vi "Module Template SM.vi"(8 "error in (no error)":errorcluster, 11 "Module_Refs":T1={"ModuleName"=enum."Controller", "Queue"=refnum, "user event"=refnum, "VI Refnum"=refnum, "ShowFP"=FALSE, "StatesTracking Enabled"=FALSE}) -> (0 "error out":errorcluster)   [LabVIEW 2019, in "Architecture.lvlib" / "Module Template.lvlib"]
doc: "Main Module Template of the architecture. Use this as a template to integrate new independent processes into your application."
uses:
  Modules/Module Template/Module Template.lvlib
  Typedefs/Module References.ctl
  Typedefs/Enum_Module_Name.ctl
  Typedefs/Message.ctl
  Typedefs/State Machine Data.ctl
  Modules/Module Template/Typedefs/Config.ctl
  Typedefs/Application Configuration.ctl
  Modules/Module Template/SubVIs/Module Template Configuraton Extractor API.vi
  Architecture.lvlib
panel:
  in  "Stop App":bool
  out "Message":string
  in  "Stop Module":bool
  # "#Architecture\n\nPlace inside this box all visible data."
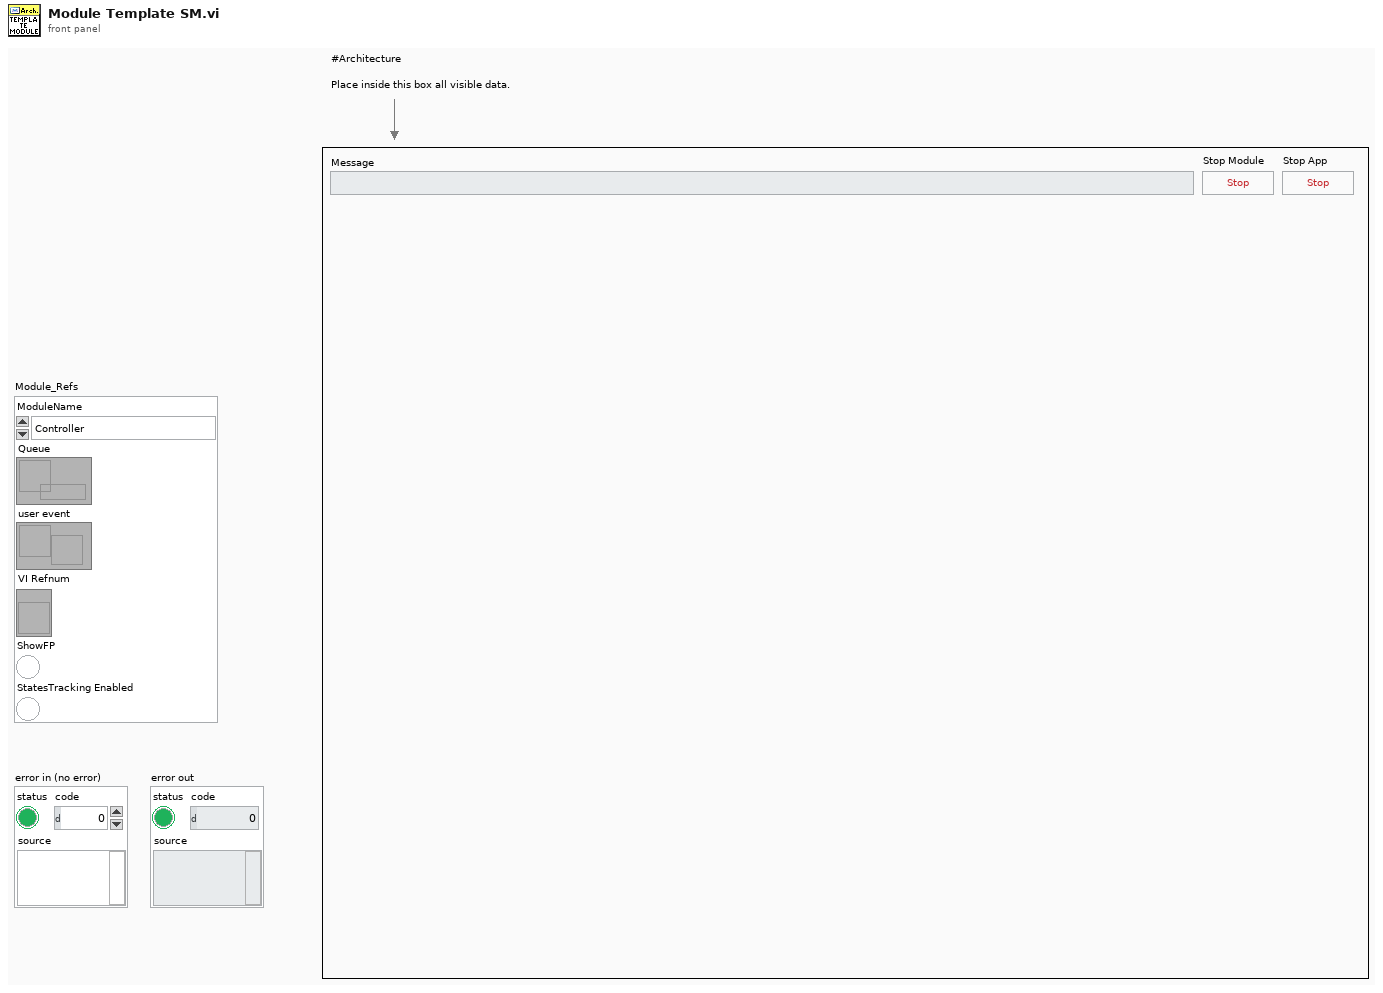
[diagram p1: front panel]
types:
  T1 = typedef "Architecture.lvlib/Module References.ctl" = cluster{"ModuleName":T2, "Queue":refnum<queue>, "user event":refnum<user-event>, "VI Refnum":refnum<vi>, "ShowFP":bool, "StatesTracking Enabled":bool}
  T2 = typedef "Architecture.lvlib/Enum_Module_Name.ctl" = enum16{"Configuration", "Error_Handler", "Log", "Database", "Controller", "User Console", "Display Console", "Sensor Interface"}
  T3 = typedef "Architecture.lvlib/Module Template.lvlib/State Machine Data.ctl" = cluster{"Module_Refs":T1, "Response Data":variant, "Module Template Config":T4}
  T4 = typedef "Architecture.lvlib/Module Template.lvlib/Config.ctl" = cluster{"Module Enabled":bool}
  T5 = enum32{"Invalid", "Standard", "Closed", "Hidden", "Minimized", "Maximized"}
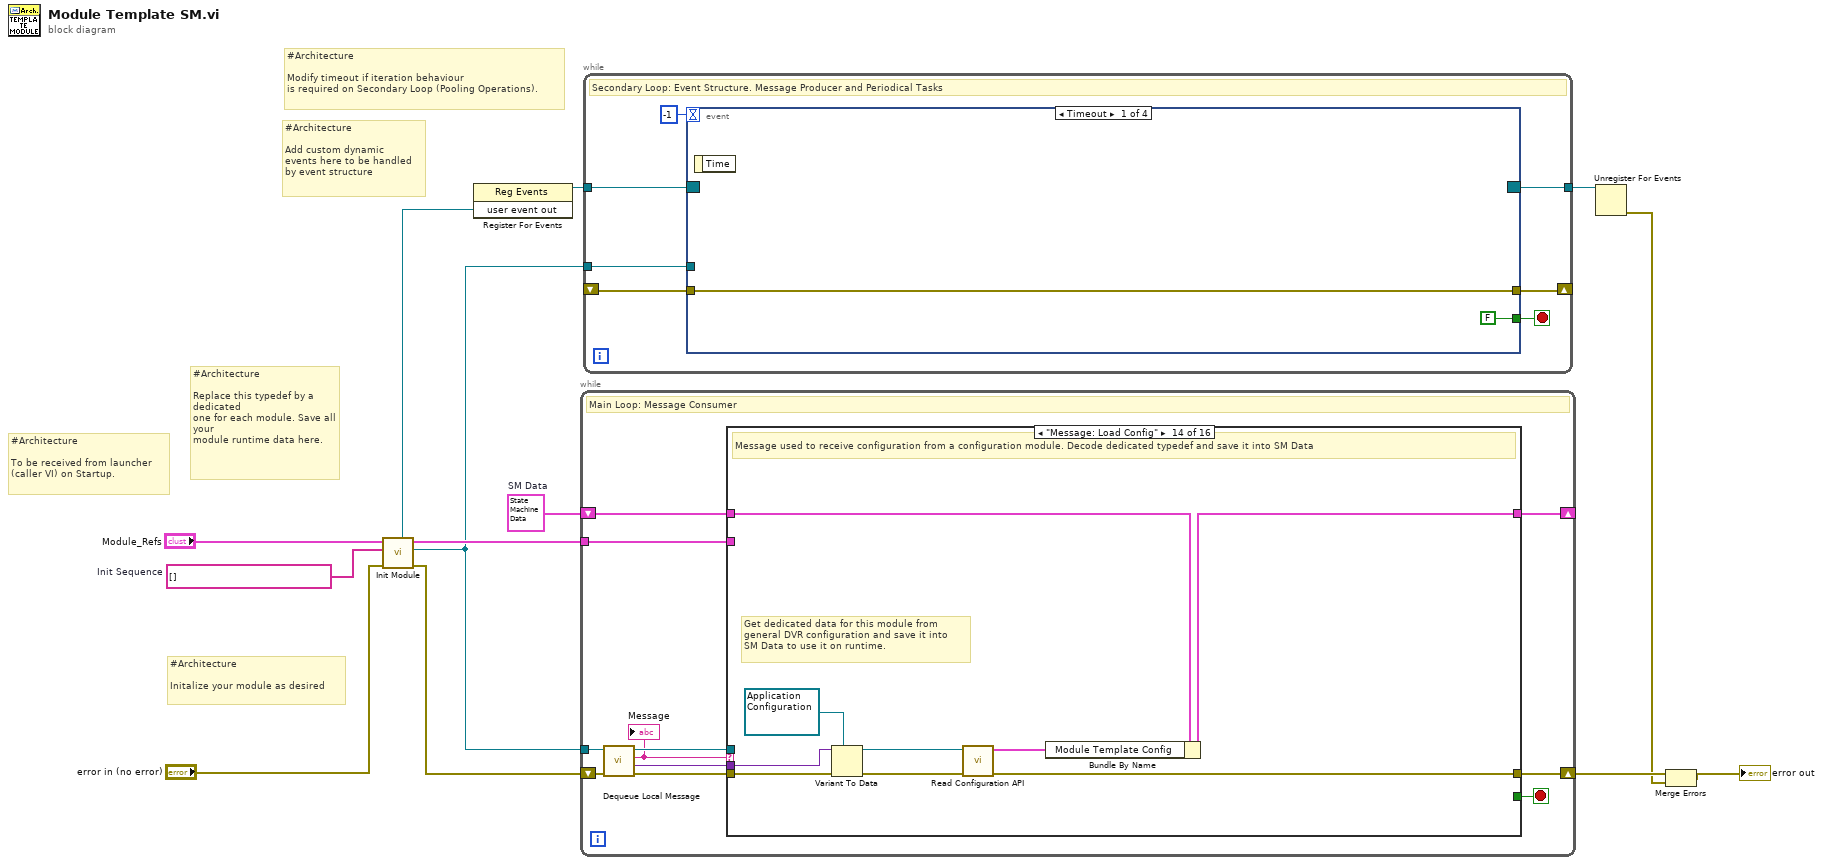
[diagram p0: block diagram]
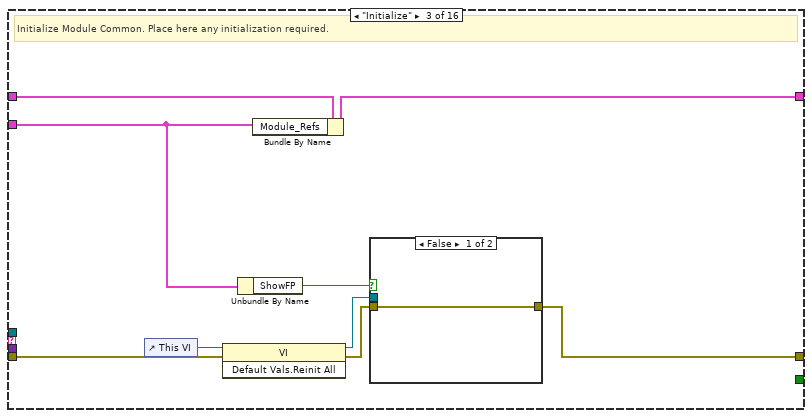
[diagram p4: hidden frame]
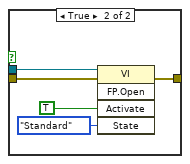
[diagram p5: hidden frame]
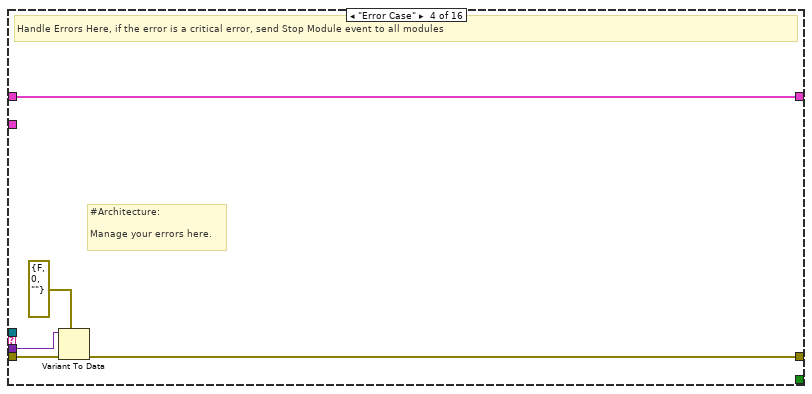
[diagram p6: hidden frame]
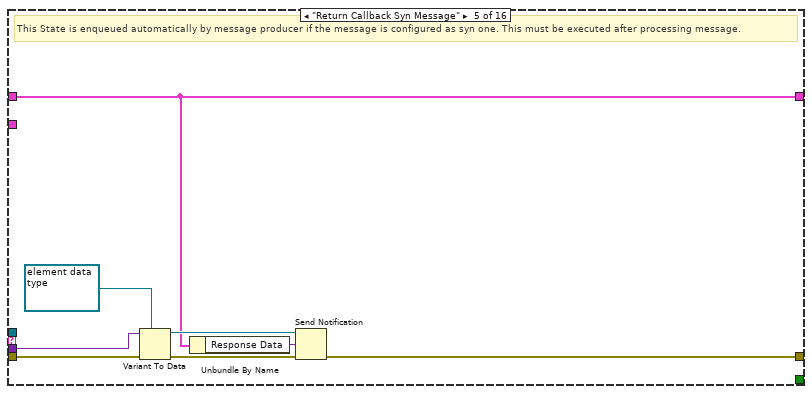
[diagram p7: hidden frame]
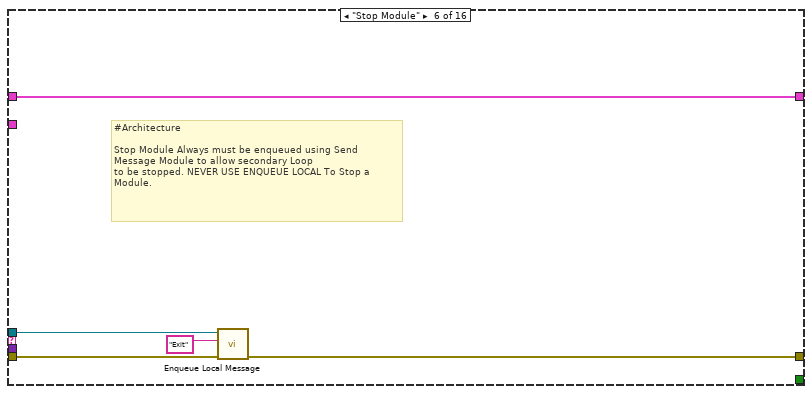
[diagram p8: hidden frame]
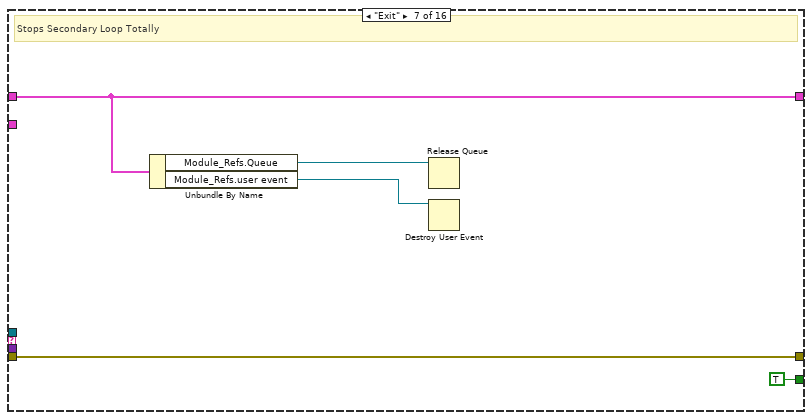
[diagram p9: hidden frame]
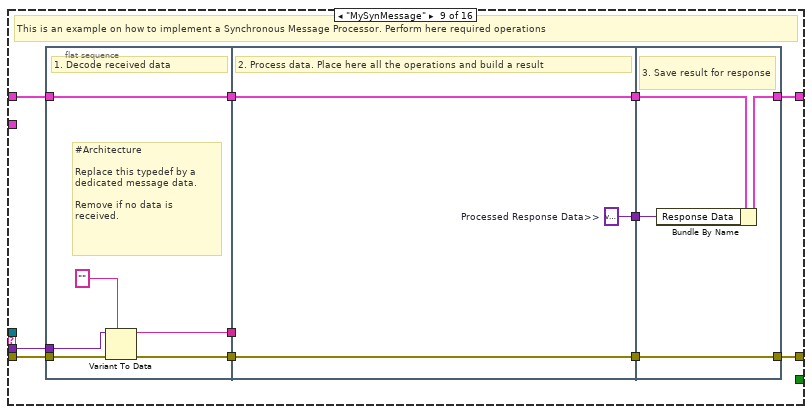
[diagram p11: hidden frame]
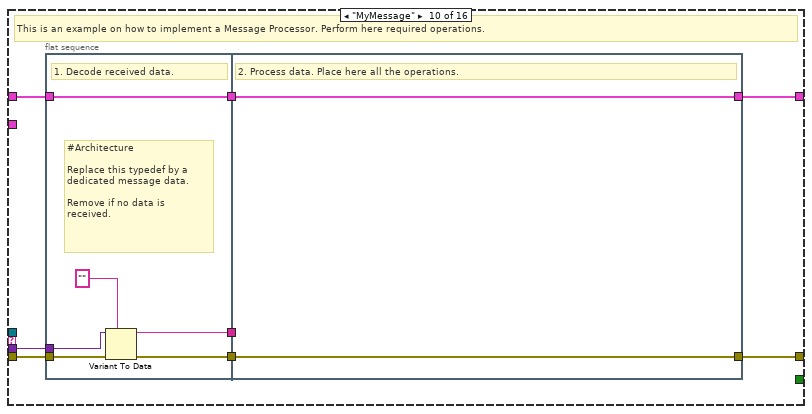
[diagram p12: hidden frame]
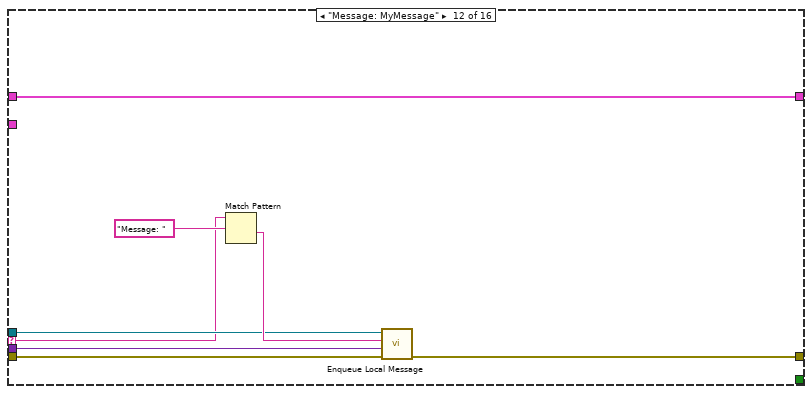
[diagram p14: hidden frame]
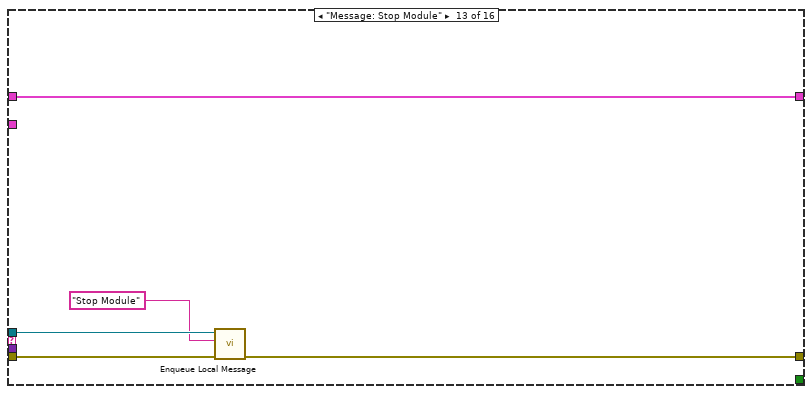
[diagram p15: hidden frame]
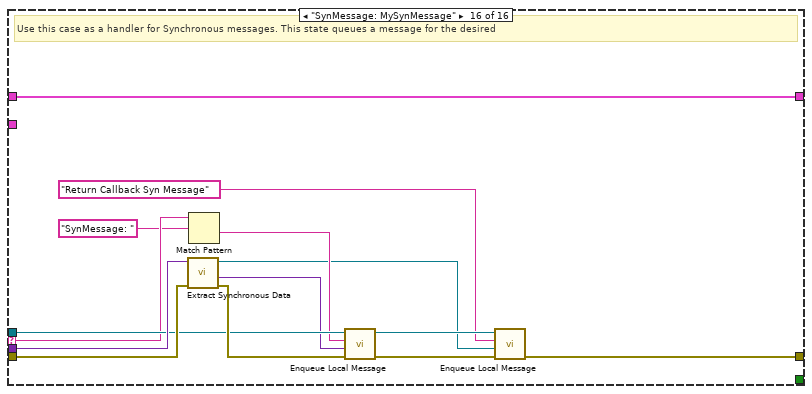
[diagram p17: hidden frame]
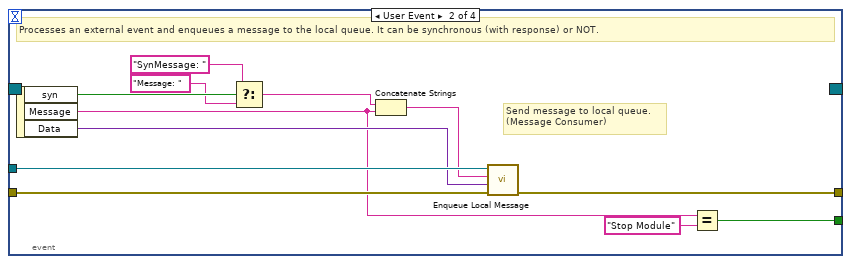
[diagram p18: hidden frame]
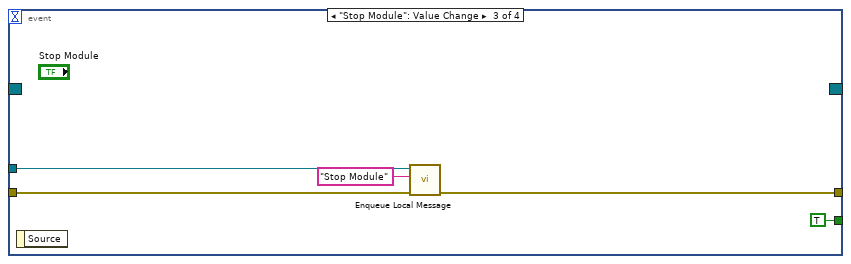
[diagram p19: hidden frame]
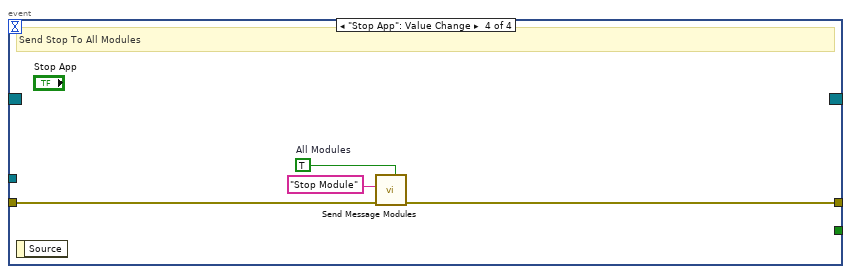
[diagram p20: hidden frame]
diagram:
  w10 = string[] []  # Init Sequence
  w13 = T3 {"Module_Refs"={"ModuleName"=enum."Controller", "Queue"=refnum, "user event"=refnum, "VI Refnum"=refnum, "ShowFP"=FALSE, "StatesTracking Enabled"=FALSE}, "Response Data"=variant, "Module Template Config"={"Module Enabled"=FALSE}}  # SM Data
  # "#Architecture\n\nModify timeout if iteration behaviour \nis required on Secondary Loop (Pooling Operations)."
  # "#Architecture\n\nAdd custom dynamic \nevents here to be handled \nby event structure"
  # "#Architecture\n\nInitalize your module as desired"
  # "#Architecture\n\nTo be received from launcher \n(caller VI) on Startup."
  # "#Architecture\n\nReplace this typedef by a dedicated \none for each module. Save all your \nmodule runtime data here."
  n1 = call "Init Module.vi"("error in (no error)"="error in (no error)", "Init Sequence"=w10, "Module Refs"="Module_Refs") -> ("error out"=w12:errorcluster, "queue out"=w1:refnum<queue>, "Module Refs Out"=w3:T1, "user event out"=w2:refnum<user-event>)  [unwired: 5 in]
  n2 = register-events(w2) -> (reference out=w9:refnum<event-registration>)  [unwired: 2 in, 1 out]
  n3 = while {
    shift-right: [w23] -> _
    shift-left: w13 -> [w24]
    shift-right: [w22] -> w7
    shift-left: w12 -> [w20]
    tunnel: w1 -> [w21]
    tunnel: w3 -> [w14]
    stop <- w15 stop-if-true
    # "Main Loop: Message Consumer"
    n4 = call "Dequeue Local Message.vi"("error in"=w20, "Msg queue in"=w21) -> ("error out"=w19:errorcluster, "Data"=w16:variant, "Message"=w17:string, "queue out"=w18:refnum<queue>)  [unwired: 6 in]
    "Message" <- w17
    n5 = case shown="\"Message: Load Config\"" w17 {
      selector: w17 -> [_ _ _ _ _ _ _ _ _ _ _ w111 _ _ _ w143]
      tunnel: w24 -> [w26 w28 w37 w48 w50 w61 w64 w68 w79 w100 w110 w118 w123 w132 w134 w148]
      tunnel: [w26 w28 w35 w48 w50 w61 w64 w68 w78 w93 w110 w118 w123 w125 w134 w148] -> w23
      tunnel: w19 -> [w25 w27 w36 w47 w56 w60 w66 w67 w72 w96 w109 w115 w122 w131 w133 w147]
      tunnel: [w25 w27 w31 w46 w55 w59 w66 w67 w77 w99 w109 w112 w121 w126 w133 w137] -> w22
      tunnel: w18 -> [_ _ _ _ _ w58 _ _ _ _ _ w113 w120 _ _ w144]
      tunnel: w16 -> [_ _ _ w45 w53 _ _ _ w71 w95 _ w114 _ w130 _ w145]
      tunnel: [_ _ _ _ _ _ TRUE _ _ _ _ _ _ _ _ _] -> w15
      tunnel: w14 -> [_ _ w34 _ _ _ _ _ _ _ _ _ _ _ _ _]
      frame "--------State Machine Arquitechture Operations--------" {
      }
      frame "Idle", Default {
        # "Use this state to make iterations if required."
      }
      frame "Initialize" {
        # "Initialize Module Common. Place here any initialization required."
        n6 = control-ref of="This VI"() -> (w29:refnum<vi>)
        n7 = invoke class="VI" method="Default Vals.Reinit All"(reference=w29, error in=w36) -> (reference out=w32:refnum<vi>, error out=w33:errorcluster)  [unwired: 1 in, 1 out]
        n8 = Unbundle By Name(w34) -> ("ShowFP"=w30:bool)
        n9 = Bundle By Name(cluster=w37, "Module_Refs"=w34) -> (w35:T3)
        n10 = case shown="False" w30 {
          tunnel: w33 -> [w38 w43]
          tunnel: [w38 w42] -> w31
          tunnel: w32 -> [_ w41]
          frame False {
          }
          frame True {
            n11 = invoke class="VI" method="FP.Open"(reference=w41, error in=w43, "Activate"=TRUE ("Activate?"), "State"=T5."Standard") -> (error out=w42:errorcluster)  [unwired: 1 in, 4 out]
          }
        }
      }
      frame "Error Case" {
        # "#Architecture: \n\nManage your errors here."
        # "Handle Errors Here, if the error is a critical error, send Stop Module event to all modules"
        n12 = Variant To Data(error in=w47, type=errorcluster {"status"=FALSE, "code"=0, "source"=""} ("error constant"), Variant=w45) -> (error out=w46:errorcluster)  [unwired: 1 out]
      }
      frame "Return Callback Syn Message" {
        # "This State is enqueued automatically by message producer if the message is configured as syn one. This must be executed after processing message."
        n13 = Variant To Data(error in=w56, type=refnum<notifier> refnum ("notifier out"), Variant=w53) -> (data=w51:refnum<notifier>, error out=w54:errorcluster)
        n14 = Unbundle By Name(w50) -> ("Response Data"=w49:variant)
        n15 = Send Notification(notification=w49, notifier=w51, error in (no error)=w54) -> (error out=w55:errorcluster)  [unwired: 1 out]
      }
      frame "Stop Module" {
        # "#Architecture\n\nStop Module Always must be enqueued using Send Message Module to allow secondary Loop\nto be stopped. NEVER USE ENQUEUE LOCAL To Stop a Module."
        n16 = call "Enqueue Local Message.vi"("error in"=w60, "Message"="Exit", "Msg queue in"=w58) -> ("error out"=w59:errorcluster)  [unwired: 7 in, 1 out]
      }
      frame "Exit" {
        # "Stops Secondary Loop Totally"
        n17 = Unbundle By Name(w64) -> ("Module_Refs.Queue"=w63:refnum<queue>, "Module_Refs.user event"=w62:refnum<user-event>)
        n18 = Release Queue(queue=w63) -> ()  [unwired: 2 in, 3 out]
        n19 = Destroy User Event(user event=w62) -> ()  [unwired: 1 in, 1 out]
      }
      frame "--------------State Machine Custom States-------------" {
      }
      frame "MySynMessage" {
        # "This is an example on how to implement a Synchronous Message Processor. Perform here required operations"
        n20 = flat-sequence {
          tunnel: w72 -> [w83]
          tunnel: w79 -> [w85]
          tunnel: [w85] -> w76
          tunnel: [w81] -> w75
          tunnel: w71 -> [w82]
          tunnel: [w80] -> w70
          tunnel: w76 -> [w88]
          tunnel: w75 -> [w87]
          tunnel: [w88] -> w74
          tunnel: [w87] -> w73
          tunnel: w70 -> [_]
          tunnel: [w86] -> w69
          tunnel: [w91] -> w77
          tunnel: [w90] -> w78
          tunnel: w74 -> [w92]
          tunnel: w73 -> [w91]
          tunnel: w69 -> [w89]
          frame #0 {
            # "#Architecture\n\nReplace this typedef by a dedicated message data.\n\nRemove if no data is received."
            # "1. Decode received data"
            n21 = Variant To Data(error in=w83, type="", Variant=w82) -> (data=w80:string, error out=w81:errorcluster)
          }
          frame #1 {
            w86 = variant  # Processed Response Data>>
            # "2. Process data. Place here all the operations and build a result"
          }
          frame #2 {
            # "3. Save result for response"
            n22 = Bundle By Name(cluster=w92, "Response Data"=w89) -> (w90:T3)
          }
        }
      }
      frame "MyMessage" {
        # "This is an example on how to implement a Message Processor. Perform here required operations."
        n23 = flat-sequence {
          tunnel: w96 -> [w104]
          tunnel: w100 -> [w106]
          tunnel: [w106] -> w98
          tunnel: [w102] -> w97
          tunnel: w95 -> [w103]
          tunnel: [w101] -> w94
          tunnel: w98 -> [w107]
          tunnel: w97 -> [w108]
          tunnel: w94 -> [_]
          tunnel: [w108] -> w99
          tunnel: [w107] -> w93
          frame #0 {
            # "#Architecture\n\nReplace this typedef by a dedicated message data.\n\nRemove if no data is received."
            # "1. Decode received data."
            n24 = Variant To Data(error in=w104, type="", Variant=w103) -> (data=w101:string, error out=w102:errorcluster)
          }
          frame #1 {
            # "2. Process data. Place here all the operations."
          }
        }
      }
      frame "--------------Dynamic Events Messages----------------" {
      }
      frame "Message: MyMessage" {
        n25 = Match Pattern(string=w111, regular expression="Message: ") -> (after substring=w116:string)  [unwired: 1 in, 3 out]
        n26 = call "Enqueue Local Message.vi"("error in"=w115, "Data"=w114, "Message"=w116, "Msg queue in"=w113) -> ("error out"=w112:errorcluster)  [unwired: 6 in, 1 out]
      }
      frame "Message: Stop Module" {
        n27 = call "Enqueue Local Message.vi"("error in"=w122, "Message"="Stop Module", "Msg queue in"=w120) -> ("error out"=w121:errorcluster)  [unwired: 7 in, 1 out]
      }
      frame "Message: Load Config" {
        # "Get dedicated data for this module from \ngeneral DVR configuration and save it into \nSM Data to use it on runtime."
        # "Message used to receive configuration from a configuration module. Decode dedicated typedef and save it into SM Data"
        n28 = Variant To Data(error in=w131, type=refnum<data-value> refnum ("data value reference"), Variant=w130) -> (data=w128:refnum<data-value>, error out=w127:errorcluster)
        n29 = call-poly "Read Configuration API.vi"("error constant"=w127, "General Config DVR In"=w128) -> ("error out"=w126:errorcluster, "Module Template Config"=w124:T4)  [unwired: 8 in]
        n30 = Bundle By Name(cluster=w132, "Module Template Config"=w124) -> (w125:T3)
      }
      frame "------------Synchronous Event Messages--------------" {
      }
      frame "SynMessage: MySynMessage" {
        # "Use this case as a handler for Synchronous messages. This state queues a message for the desired"
        n31 = call "Extract Synchronous Data.vi"("error in 2"=w147, "Variant"=w145) -> ("error in"=w146:errorcluster, "Data Out"=w140:variant, "notifier out"=w135:refnum<notifier>)  [unwired: 7 in]
        n32 = Match Pattern(string=w143, regular expression="SynMessage: ") -> (after substring=w141:string)  [unwired: 1 in, 3 out]
        n33 = call "Enqueue Local Message.vi"("error in"=w146, "Data"=w140, "Message"=w141, "Msg queue in"=w144) -> ("error out"=w139:errorcluster, "queue out"=w138:refnum<queue>)  [unwired: 6 in]
        n34 = call "Enqueue Local Message.vi"("error in"=w139, "Data"=w135, "Message"="Return Callback Syn Message", "Msg queue in"=w138) -> ("error out"=w137:errorcluster)  [unwired: 6 in, 1 out]
      }
    }
  }
  n35 = while {
    tunnel: w9 -> [w155]
    tunnel: w1 -> [w152]
    tunnel: [w151] -> w8
    shift-right: [w149] -> _
    shift-left: _ -> [w150]
    stop <- w153 stop-if-true
    # "Secondary Loop: Event Structure. Message Producer and Periodical Tasks"
    n36 = event shown="[0] Timeout" {
      selector: w155 -> [_ _ _ _]
      dyn-events: [_ _ _ _] -> w151
      timeout: -1 -> [_ _ _ _]
      tunnel: [FALSE w164 TRUE _] -> w153
      tunnel: w152 -> [_ w169 w171 _]
      tunnel: w150 -> [w156 w168 w174 w176]
      tunnel: [w156 w167 w172 w175] -> w149
      event Timeout {
        n37 = event-data() -> ()  [unwired: 1 in, 1 out]
      }
      event User Event {
        # "Send message to local queue. \n(Message Consumer)"
        # "Processes an external event and enqueues a message to the local queue. It can be synchronous (with response) or NOT."
        n38 = event-data() -> ("syn"=w161:bool, "Message"=w163:string, "Data"=w166:variant)  [unwired: 1 in]
        n39 = Select(t="SynMessage: " ("string"), s=w161, f="Message: " ("string")) -> (s? t:f=w158:string)
        n40 = Concatenate Strings(w158, w163) -> (w165:string)
        n41 = call "Enqueue Local Message.vi"("error in"=w168, "Data"=w166, "Message"=w165, "Msg queue in"=w169) -> ("error out"=w167:errorcluster)  [unwired: 6 in, 1 out]
        n42 = Equal?(x=w163, y="Stop Module") -> (x = y?=w164:bool)
      }
      event "Stop Module": Value Change {
        n43 = event-data() -> ()  [unwired: 1 in, 1 out]
        n44 = call "Enqueue Local Message.vi"("error in"=w174, "Message"="Stop Module", "Msg queue in"=w171) -> ("error out"=w172:errorcluster)  [unwired: 7 in, 1 out]
      }
      event "Stop App": Value Change {
        w178 = TRUE  # All Modules
        # "Send Stop To All Modules"
        n45 = event-data() -> ()  [unwired: 1 in, 1 out]
        n46 = call "Send Message Modules.vi"("All Modules"=w178, "Error In"=w176, "Message"="Stop Module") -> ("error in (no error)"=w175:errorcluster)  [unwired: 8 in]
      }
    }
  }
  n47 = Unregister For Events(event registration refnum=w8) -> (error out=w6:errorcluster)  [unwired: 1 in]
  n48 = Merge Errors(w7, w6) -> (→"error out":errorcluster)
